vi "Table Contents.vi"(7 "bookmark (word)":string, 8 "error in (no error)":errorcluster, 11 "report in":refnum<class "NI_report.lvclass">) -> (0 "error out":errorcluster, 2 "table contents":string[][](array[string]), 3 "report out":refnum<class "NI_report.lvclass">)   [LabVIEW 2018, in "WordReportGeneration.lvlib" / "Word_Report.lvclass"]
uses:
  Word_Report.lvclass
  <vilib>/Utility/NIReport.llb/NI_report.lvclass
  <vilib>/Utility/NIReport.llb/Word/NI_Word.lvclass
  WordReportGeneration.lvlib
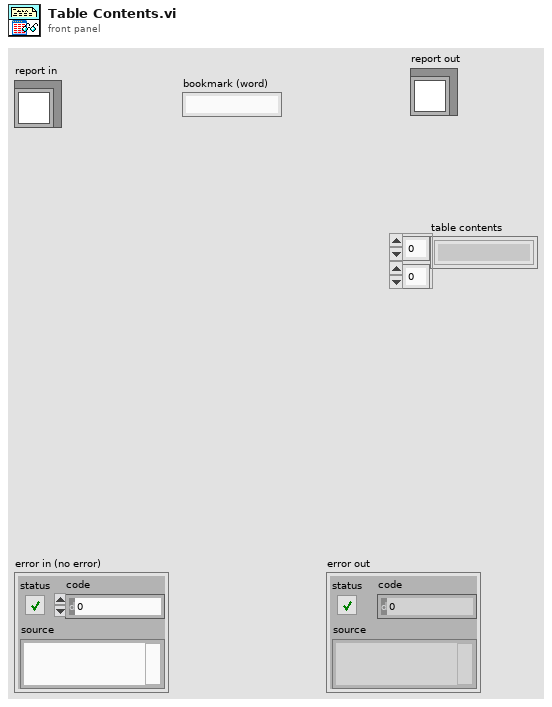
[diagram p1: front panel]
types:
  T1 = cluster{"position (Excel)":cluster{"row":i32, "column":i32}, "name (Excel) ":string, "bookmark (Word)":string}
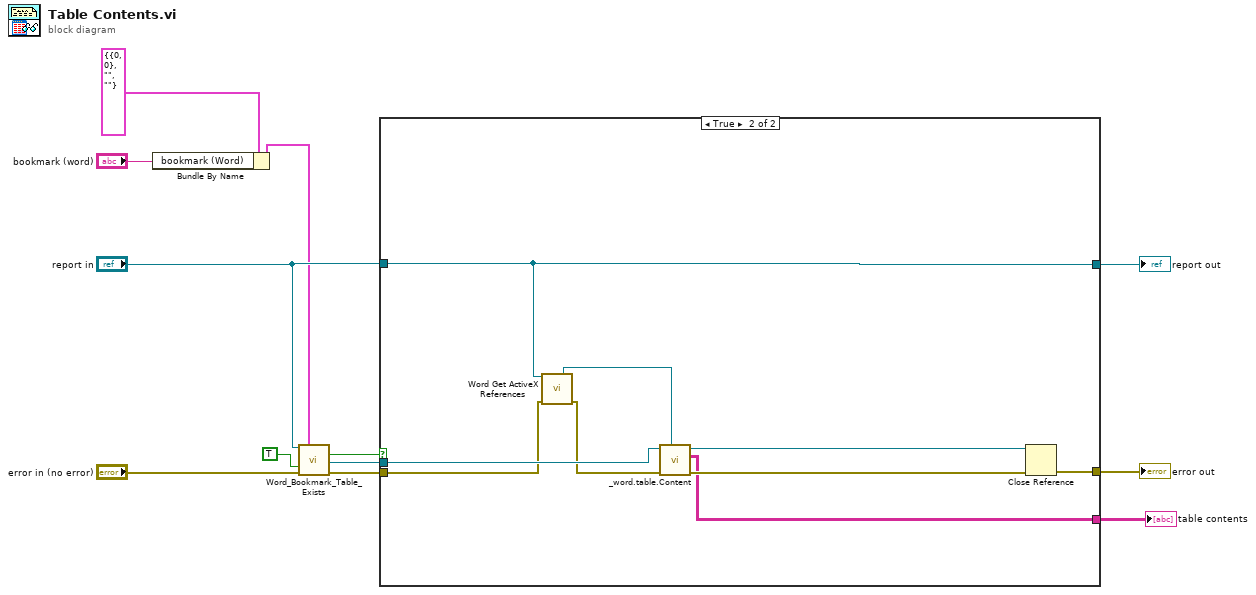
[diagram p0: block diagram]
diagram:
  n1 = Bundle By Name(cluster=T1 {"position (Excel)"={"row"=0, "column"=0}, "name (Excel) "="", "bookmark (Word)"=""} ("MS Office parameters"), "bookmark (Word)"="bookmark (word)") -> (w5:T1)
  n2 = call <vilib>:"Word_Bookmark_Table_Exists.vi"("report in"="report in", "MS Office parameters"=w5, "get table ref?"=TRUE, "error in (no error)"="error in (no error)") -> ("bookmark to existing table?"=w3:bool, "table ref"=w8:refnum<k7>, "error out"=w9:errorcluster)  [unwired: 8 in, 1 out]
  n3 = case shown="True" w3 {
    tunnel: "report in" -> [w13 w19]
    tunnel: [w14 w23] -> w11
    tunnel: w8 -> [_ w22]
    tunnel: w9 -> [w14 w17]
    tunnel: [w13 w19] -> w2
    tunnel: [_ w15] -> w1
    frame False {
    }
    frame True {
      n4 = call <vilib>:"Word Get ActiveX References.vi"("report in"=w19, "error in (no error)"=w17) -> ("Word._Application"=w18:refnum<k7>, "error out"=w16:errorcluster)  [unwired: 7 in, 5 out]
      n5 = call "_word.table.Content.vi"("word.application"=w18, "error in (no error)"=w16, "table in"=w22) -> ("error out"=w21:errorcluster, "table row contents"=w15:string[][], "table out"=w20:refnum<k7>)  [unwired: 6 in]
      n6 = Close Reference(reference=w20, error in (no error)=w21) -> (error out=w23:errorcluster)
    }
  }
  "error out" <- w11
  "report out" <- w2
  "table contents" <- w1
